vi "PID Table (Cohen-Coon).vi"(7 "Type of Controller":u16(ring) items=["P", "PI", "PID", "PD"], 9 "Dead Time (L)":dbl, 10 "Time Constant (T)":dbl, 11 "Plant Gain (K)":dbl) -> (1 "Derivative Time (Td)":dbl, 2 "Integral Time (Ti)":dbl, 3 "Proportional Gain (Kp)":dbl)   [LabVIEW 2020, in "NI_PID_autopid.lvlib"]
uses:
  <vilib>/addons/control/pid/NI_PID_autopid.lvlib
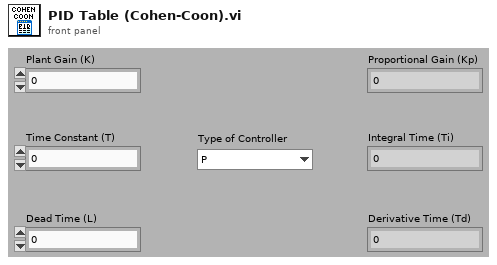
[diagram p1: front panel]
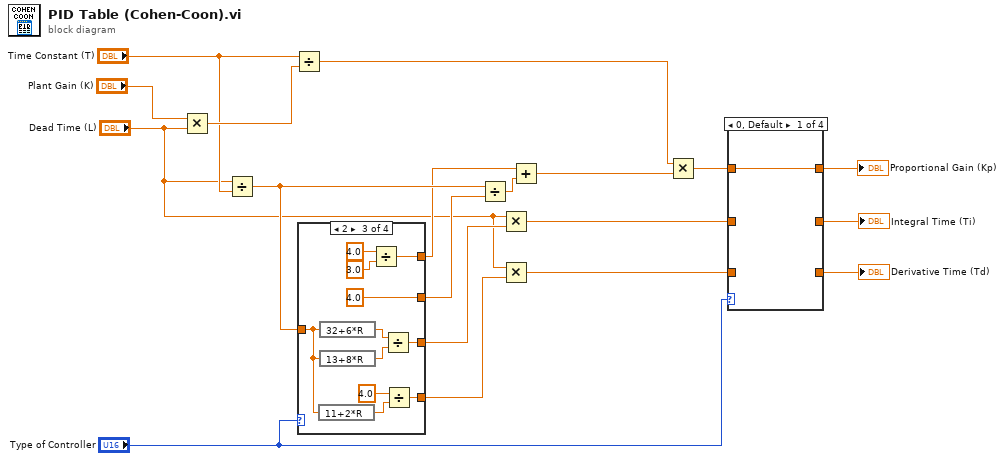
[diagram p0: block diagram]
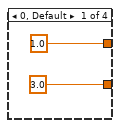
[diagram p2: hidden frame]
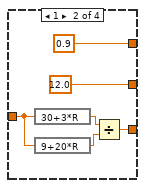
[diagram p3: hidden frame]
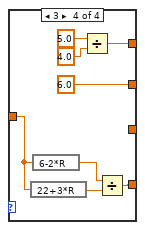
[diagram p4: hidden frame]
diagram:
  n1 = Multiply(x="Plant Gain (K)", y="Dead Time (L)") -> (x*y=w19:dbl)
  n2 = Divide(x="Dead Time (L)", y="Time Constant (T)") -> (x/y=w16:dbl)
  n3 = Divide(x="Time Constant (T)", y=w19) -> (x/y=w11:dbl)
  n4 = case shown="2" "Type of Controller" {
    tunnel: [1.0 ("Kp 6") 0.9 ("Kp 6") w30 w41] -> w9
    tunnel: [3.0 ("Kp 6") 12.0 ("Kp 6") 4.0 ("Kp 6") 6.0 ("Kp 6")] -> w18
    tunnel: w16 -> [_ w22 w32 w43]
    tunnel: [_ w23 w34 _] -> w15
    tunnel: [_ _ w31 w42] -> w13
    frame 0, Default {
    }
    frame 1 {
      n5 = expression code="30+3*R"(w22) -> (w25:dbl)
      n6 = expression code="9+20*R"(w22) -> (w24:dbl)
      n7 = Divide(x=w25, y=w24) -> (x/y=w23:dbl)
    }
    frame 2 {
      n8 = expression code="11+2*R"(w32) -> (w33:dbl)
      n9 = expression code="32+6*R"(w32) -> (w36:dbl)
      n10 = expression code="13+8*R"(w32) -> (w35:dbl)
      n11 = Divide(x=4.0 ("Kp 6"), y=3.0 ("Kp 6")) -> (x/y=w30:dbl)
      n12 = Divide(x=w36, y=w35) -> (x/y=w34:dbl)
      n13 = Divide(x=4.0, y=w33) -> (x/y=w31:dbl)
    }
    frame 3 {
      n14 = expression code="22+3*R"(w43) -> (w44:dbl)
      n15 = expression code="6-2*R"(w43) -> (w39:dbl)
      n16 = Divide(x=5.0 ("Kp 6"), y=4.0 ("Kp 6")) -> (x/y=w41:dbl)
      n17 = Divide(x=w39, y=w44) -> (x/y=w42:dbl)
    }
  }
  n18 = Divide(x=w16, y=w18) -> (x/y=w8:dbl)
  n19 = Multiply(x="Dead Time (L)", y=w15) -> (x*y=w14:dbl)
  n20 = Multiply(x="Dead Time (L)", y=w13) -> (x*y=w12:dbl)
  n21 = Add(x=w9, y=w8) -> (x+y=w10:dbl)
  n22 = Multiply(x=w11, y=w10) -> (x*y=w17:dbl)
  n23 = case shown="0, Default" "Type of Controller" {
    tunnel: w17 -> [w47 w49 w52 w54]
    tunnel: [w47 w49 w52 w54] -> w7
    tunnel: [_ w48 w50 _] -> w1
    tunnel: w14 -> [_ w48 w50 _]
    tunnel: w12 -> [_ _ w51 w53]
    tunnel: [_ _ w51 w53] -> w2
    frame 0, Default {
    }
    frame 1 {
    }
    frame 2 {
    }
    frame 3 {
    }
  }
  "Proportional Gain (Kp)" <- w7
  "Integral Time (Ti)" <- w1
  "Derivative Time (Td)" <- w2
